vi "createMessages.vi"(8 "error in (no error)":errorcluster, 10 "Messages Table":string[][](table)=[["welcome", "Welcome\r\nto\r\nLabVIEW Simon\r\nby\r\nFelipe Flores\r\n", "25", "Center", "LineByLine"], ["instructions", "\n\nSlide \"LEVEL\" to see how good you are.\n\nPress \"PLAY\" to start playing.\n\nPress \"LONGEST\" to see the longest sequence ever played.", "16", "Center", "Plain"], ["stageUp", "\\n\\rStage\\s%d", "60", "Center", "Rotate"], ["startGame", "\nLet's do it!", "40", "Center", "Plain"], ["last", "\nPlaying last Sequence...", "40", "Left", "Plain"], ["longest", "\nPlaying longest Sequence...", "40", "Left", "Plain"], ["hsHeaders", "High,Scores\r\n=========,=========\r\n", "25", "Center", "LineByLine"], ["levelChoice", "Level %d selected", "", "Left", "Plain"], ["yourTurn", "\n\nyour turn!", "40", "Center", "Plain"], ["gameTitle", "Simon Game", "10", "Left", "TitleBar"], ["playerName", "%s is playing now!", "10", "Left", "TitleBar"], ["", "", "", "", ""]]) -> (0 "error out":errorcluster, 3 "simonMessages out":refnum<class "simonMessages.lvclass">)   [LabVIEW 2019, in "simonMessages.lvclass"]
uses:
  simonMessages.lvclass
  simonMessages.lvclass/simonMessages.ctl
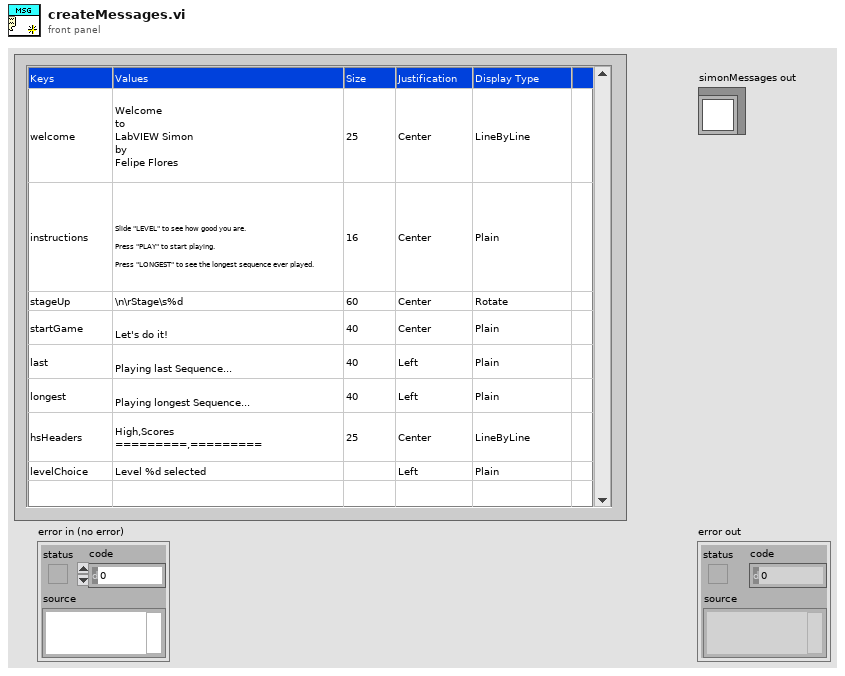
[diagram p1: front panel]
types:
  T1 = map{string, cluster{"Text":string, "Size":u8, "Justification":enum16{"Left", "Center", "Right"}, "Display Type":string}}
  T2 = cluster{"Text":string, "Size":u8, "Justification":enum16{"Left", "Center", "Right"}, "Display Type":string}
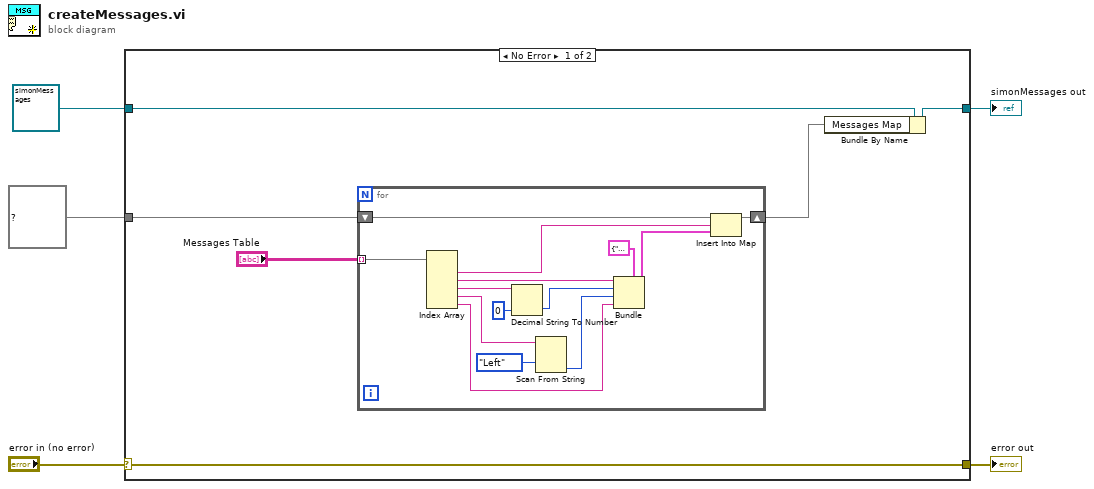
[diagram p0: block diagram]
diagram:
  n1 = case shown="No Error" "error in (no error)" {
    selector: "error in (no error)" -> [w11 w27]
    tunnel: [w11 w27] -> w4
    tunnel: [w7 w26] -> w2
    tunnel: refnum<class "simonMessages.lvclass"> refnum ("simonMessages in") -> [w10 w26]
    tunnel: T1 {} ("Messages Map") -> [w9 _]
    frame No Error {
      n2 = for {
        shift-right: [w24] -> w6
        shift-left: w9 -> [w25]
        tunnel: "Messages Table" -> [w22] mode=indexing
        n3 = Index Array(array=w22) -> (element #1=w13:string, element #2=w21:string, element #3=w20:string, element #4=w16:string, element #5=w14:string)  [unwired: 5 in]
        n4 = Decimal String To Number(string=w20, default (0L)=u8 0 ("default (0 I32)")) -> (number=w19:u8)  [unwired: 1 in, 1 out]
        n5 = Scan From String(input string=w16, default 1=enum16{"Left", "Center", "Right"}."Left" ("Justification")) -> (output 1=w15:enum16{"Left", "Center", "Right"})  [unwired: 3 in, 3 out]
        n6 = Bundle(cluster=T2 {"Text"="", "Size"=0, "Justification"=enum."Left", "Display Type"=""} ("value"), "Text"=w21, "Size"=w19, "Justification"=w15, "Display Type"=w14) -> (w23:T2)
        n7 = Insert Into Map(map in=w25, key=w13, value=w23) -> (map out=w24:T1)  [unwired: 2 out]
      }
      n8 = Bundle By Name(cluster=w10, "Messages Map"=w6) -> (w7:refnum<class "simonMessages.lvclass">)
    }
    frame Error {
    }
  }
  "error out" <- w4
  "simonMessages out" <- w2
